vi "LHF.DB.Mongo.Util.BSONEnumToStringArray.vi"(0 "BsonENUM":refnum<k24>, 1 "Extract _id":bool, 5 "error in (no error)":errorcluster) -> (14 "Documents":string[](array[string]), 15 "_id Array":string[](array[string]), 19 "error out":errorcluster)   [LabVIEW 2013, in "LHF.DB.Mongo.lvclass"]
uses:
  LHF.DB.Mongo.lvclass
  C:/Users/Ricardo/Desktop/Projetos/LabVIEW-MongoDB/src/Driver/MongoDB.Bson.dll
  LabVIEW-MongoDB/src/Driver/MongoDB.Bson.dll
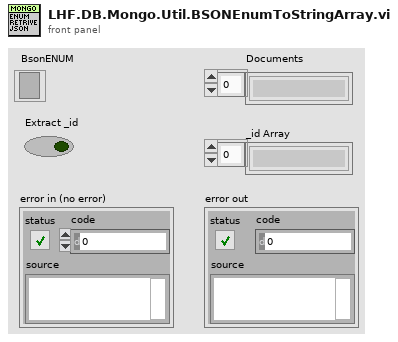
[diagram p1: front panel]
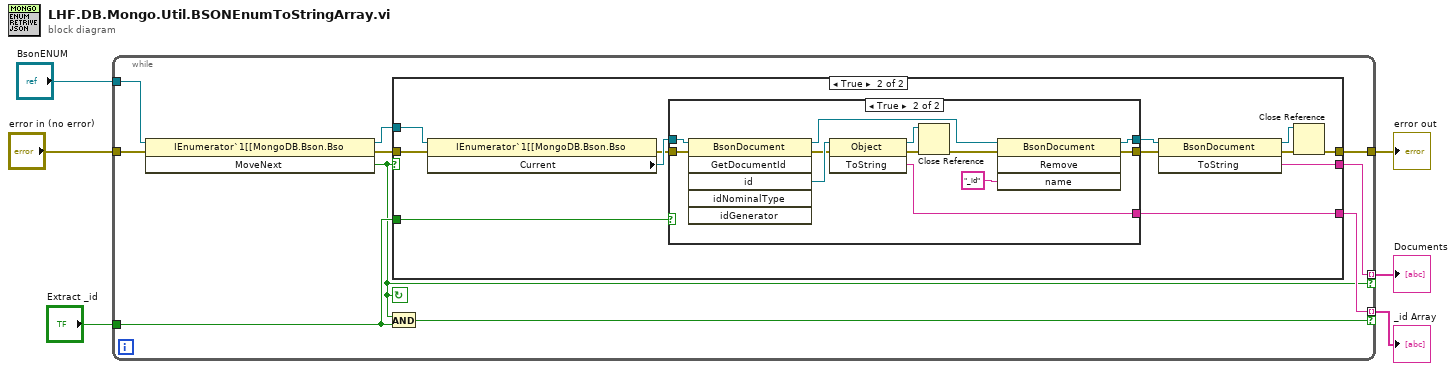
[diagram p0: block diagram]
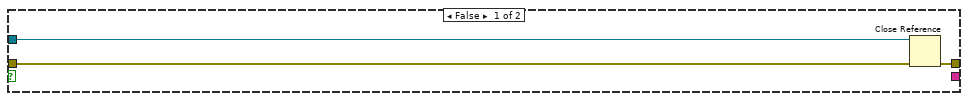
[diagram p2: hidden frame]
diagram:
  n1 = while {
    tunnel: [w14] -> w2 mode=indexing if=w8
    tunnel: [w12] -> w4
    tunnel: "error in (no error)" -> [w11]
    tunnel: "BsonENUM" -> [w16]
    tunnel: [w10] -> w5 mode=indexing if=w7
    tunnel: "Extract _id" -> [w9]
    stop <- w8 continue-if-true
    n2 = invoke class="IEnumerator`1[[MongoDB.Bson.Bso" method="MoveNext"(reference=w16, error in=w11) -> (reference out=w15:refnum<k24>, error out=w13:errorcluster, "MoveNext"=w8:bool)  [unwired: 1 in]
    n3 = And(x=w8, y=w9) -> (x .and. y?=w7:bool)
    n4 = case shown="True" w8 {
      tunnel: w15 -> [w18 w31]
      tunnel: [_ w30] -> w14
      tunnel: w13 -> [w19 w29]
      tunnel: [w17 w28] -> w12
      tunnel: [_ w27] -> w10
      tunnel: w9 -> [_ w21]
      frame False {
        n5 = Close Reference(reference=w18, error in (no error)=w19) -> (error out=w17:errorcluster)
      }
      frame True {
        n6 = property class="IEnumerator`1[[MongoDB.Bson.Bso"(reference=w31, error in=w29) -> (error out=w24:errorcluster, "Current"=w26:refnum<k24>)  [unwired: 1 out]
        n7 = case shown="True" w21 {
          tunnel: [_ w44] -> w27
          tunnel: w26 -> [w33 w42]
          tunnel: [w33 w41] -> w25
          tunnel: w24 -> [w32 w40]
          tunnel: [w32 w38] -> w22
          frame False {
          }
          frame True {
            n8 = invoke class="BsonDocument" method="GetDocumentId"(reference=w42, error in=w40) -> (reference out=w39:refnum<k24>, error out=w43:errorcluster, "id"=w45:refnum<k24>)  [unwired: 4 in, 3 out]
            n9 = invoke class="Object" method="ToString"(reference=w45, error in=w43) -> (reference out=w36:refnum<k24>, error out=w35:errorcluster, "ToString"=w44:string)  [unwired: 1 in]
            n10 = Close Reference(reference=w36, error in (no error)=w35) -> (error out=w34:errorcluster)
            n11 = invoke class="BsonDocument" method="Remove"(reference=w39, error in=w34, "name"="_id") -> (reference out=w41:refnum<k24>, error out=w38:errorcluster)  [unwired: 1 in, 2 out]
          }
        }
        n12 = invoke class="BsonDocument" method="ToString"(reference=w25, error in=w22) -> (reference out=w23:refnum<k24>, error out=w20:errorcluster, "ToString"=w30:string)  [unwired: 1 in]
        n13 = Close Reference(reference=w23, error in (no error)=w20) -> (error out=w28:errorcluster)
      }
    }
  }
  "_id Array" <- w5
  "error out" <- w4
  "Documents" <- w2
